vi "LoadSubpanelsIntoMemory.vi"(8 "error in (no error)":errorcluster, 11 "EmbeddedMainUI in":refnum<class "EmbeddedMainUI.lvclass">) -> (0 "error out":errorcluster, 3 "EmbeddedMainUI out":refnum<class "EmbeddedMainUI.lvclass">)   [LabVIEW 2016, in "EmbeddedMainUI.lvclass"]
uses:
  EmbeddedMainUI.lvclass
  <vilib>/Levylab/Embedded SMO UI/EmbeddedSMO.lvclass
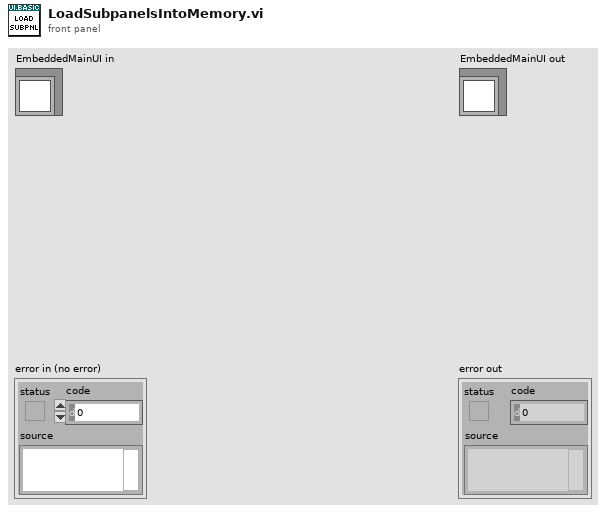
[diagram p1: front panel]
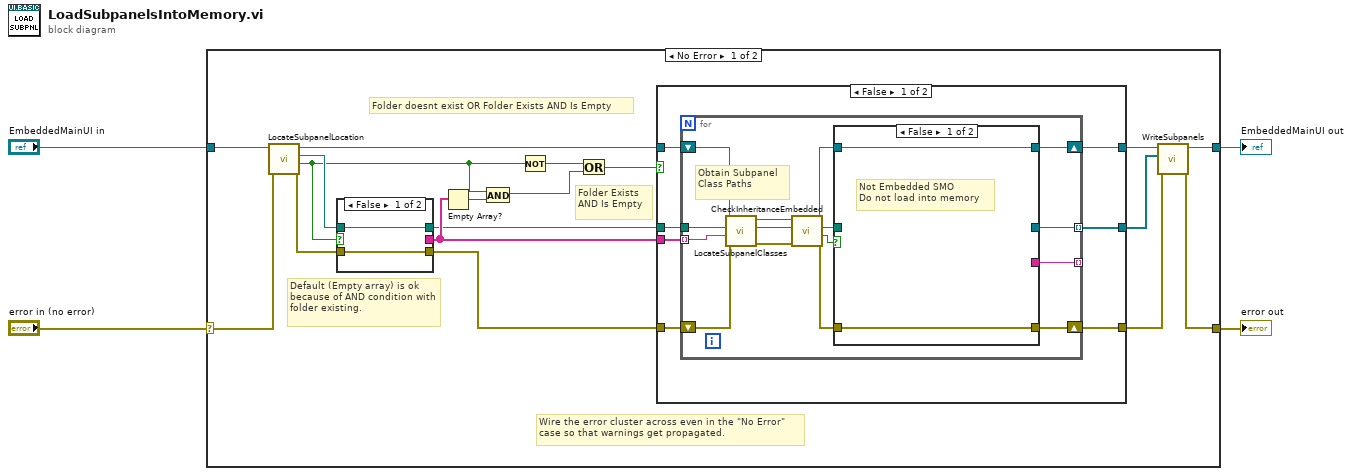
[diagram p0: block diagram]
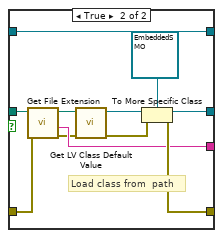
[diagram p2: hidden frame]
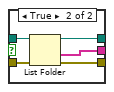
[diagram p4: hidden frame]
diagram:
  n1 = case shown="No Error" "error in (no error)" {
    selector: "error in (no error)" -> [w9 w69]
    tunnel: [w7 w69] -> w3
    tunnel: [w6 w68] -> w1
    tunnel: "EmbeddedMainUI in" -> [w8 w68]
    frame No Error {
      # "Folder doesnt exist OR Folder Exists AND Is Empty"
      # "Default (Empty array) is ok because of AND condition with folder existing."
      # "Folder Exists AND Is Empty"
      # "Wire the error cluster across even in the \"No Error\"\ncase so that warnings get propagated."
      n2 = call "LocateSubpanelLocation.vi"("error in (no error)"=w9, "EmbeddedMainUI in"=w8) -> ("error out"=w21:errorcluster, "Folder Exists?"=w18:bool, "Folder Location"=w22:path, "EmbeddedMainUI out"=w12:refnum<class "EmbeddedMainUI.lvclass">)  [unwired: 6 in]
      n3 = case shown="False" w18 {
        tunnel: w22 -> [w62 w67]
        tunnel: w21 -> [w61 w66]
        tunnel: [w62 w65] -> w14
        tunnel: [w61 w63] -> w13
        tunnel: [_ w64] -> w15
        frame False {
        }
        frame True {
          n4 = List Folder(path=w67, error in=w66) -> (path out=w65:path, folder names=w64:string[], error out=w63:errorcluster)  [unwired: 2 in, 1 out]
        }
      }
      n5 = Empty Array?(array=w15) -> (empty?=w20:bool)
      n6 = And(x=w18, y=w20) -> (x .and. y?=w19:bool)
      n7 = Not(x=w18) -> (.not. x?=w17:bool)
      n8 = Or(x=w17, y=w19) -> (x .or. y?=w16:bool)
      n9 = case shown="False" w16 {
        tunnel: w15 -> [w28 _]
        tunnel: w14 -> [w29 _]
        tunnel: w13 -> [w27 w60]
        tunnel: [w26 w60] -> w10
        tunnel: [w25 refnum<class "EmbeddedSMO.lvclass">[] []] -> w5
        tunnel: w12 -> [w24 w58]
        tunnel: [w23 w58] -> w11
        frame False {
          n10 = for {
            tunnel: w29 -> [w40]
            tunnel: w28 -> [w39] mode=indexing
            tunnel: [w44] -> w25 mode=indexing
            shift-right: [w43] -> w26
            shift-left: w27 -> [w37]
            tunnel: [w42] -> _ mode=indexing
            shift-right: [w41] -> w23
            shift-left: w24 -> [w38]
            # "Obtain Subpanel Class Paths"
            n11 = call "LocateSubpanelClasses.vi"("error in (no error)"=w37, "Folder Name"=w39, "Base Path"=w40, "EmbeddedMainUI in"=w38) -> ("error out"=w33:errorcluster, "Class Path"=w35:path, "EmbeddedMainUI out"=w34:refnum<class "EmbeddedMainUI.lvclass">)  [unwired: 5 in]
            n12 = call "CheckInheritanceEmbedded.vi"("error in (no error)"=w33, "Class Path"=w35, "EmbeddedMainUI in"=w34) -> ("error out"=w32:errorcluster, "Embedded SMO?"=w30:bool, "Class Path"=w31:path, "EmbeddedMainUI out"=w36:refnum<class "EmbeddedMainUI.lvclass">)  [unwired: 5 in]
            n13 = case shown="False" w30 {
              tunnel: [_ w57] -> w44
              tunnel: w32 -> [w46 w50]
              tunnel: [w46 w53] -> w43
              tunnel: [_ w51] -> w42
              tunnel: [w45 w48] -> w41
              tunnel: w36 -> [w45 w48]
              tunnel: w31 -> [_ w47]
              frame False {
                # "Not Embedded SMO\nDo not load into memory"
              }
              frame True {
                # "Load class from  path"
                n14 = call <vilib>:"Get File Extension.vi"("error in (no error)"=w50, "file"=w47) -> ("error out"=w49:errorcluster, "filename without extension"=w51:string, "dup file"=w52:path)  [unwired: 5 in, 2 out]
                n15 = call <vilib>:"Get LV Class Default Value.vi"("error in (no error)"=w49, "class path"=w52) -> ("error out"=w54:errorcluster, "object"=w56:refnum<class>)  [unwired: 8 in]
                n16 = To More Specific Class(target class=refnum<class "EmbeddedSMO.lvclass"> refnum ("EmbeddedSMO"), reference=w56, error in=w54) -> (specific class reference=w57:refnum<class "EmbeddedSMO.lvclass">, error out=w53:errorcluster)
              }
            }
          }
        }
        frame True {
        }
      }
      n17 = call "WriteSubpanels.vi"("error in (no error)"=w10, "Subpanels"=w5, "EmbeddedMainUI in"=w11) -> ("error out"=w7:errorcluster, "EmbeddedMainUI out"=w6:refnum<class "EmbeddedMainUI.lvclass">)  [unwired: 7 in]
    }
    frame Error {
    }
  }
  "error out" <- w3
  "EmbeddedMainUI out" <- w1
